vi "read_params.vi"(8 "error in (no error)":errorcluster, 11 "MeanShift in":refnum<class "MeanShift.lvclass">) -> (0 "error out":errorcluster, 2 "params":T1={"bandwidth"={"bandwidth_type"="None", "bandwidth_float"=0.0}, "seeds"={"seeds_type"="None", "seeds_list"=[]}, "bin_seeding"=FALSE, "min_bin_freq"=1.0, "cluster_all"=TRUE, "n_jobs"=1.0, "max_iter"=300.0}, 3 "MeanShift out":refnum<class "MeanShift.lvclass">)   [LabVIEW 2020, in "MeanShift.lvclass"]
uses:
  MeanShift.lvclass
  Controls/mean_shift_params.ctl
  MeanShift.lvclass/MeanShift.ctl
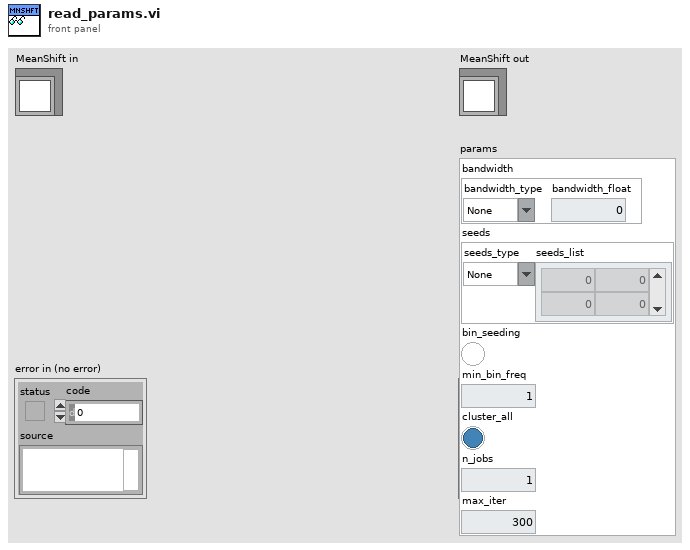
[diagram p1: front panel]
types:
  T1 = typedef "mean_shift_params.ctl" = cluster{"bandwidth":cluster{"bandwidth_type":string, "bandwidth_float":dbl}, "seeds":cluster{"seeds_type":string, "seeds_list":dbl[][]}, "bin_seeding":bool, "min_bin_freq":dbl, "cluster_all":bool, "n_jobs":dbl, "max_iter":dbl}
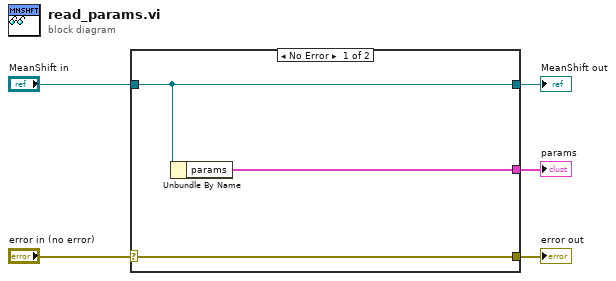
[diagram p0: block diagram]
diagram:
  n1 = case shown="No Error" "error in (no error)" {
    selector: "error in (no error)" -> [w8 w9]
    tunnel: [w8 w9] -> w4
    tunnel: [w7 w10] -> w2
    tunnel: "MeanShift in" -> [w7 w10]
    tunnel: [w6 _] -> w1
    frame No Error {
      n2 = Unbundle By Name(w7) -> ("params"=w6:T1)
    }
    frame Error {
    }
  }
  "error out" <- w4
  "MeanShift out" <- w2
  "params" <- w1
